vi "Label Example modified3.vi"() -> ()   [LabVIEW 2016]
doc: "This example shows how to label a binary image that contains multiple particles. The labeling process assigns a unique value to all the pixels that belong to a particle. Some processing functions in NI Vision require the input binary image to be labeled."
uses:
  <vilib>/vision/NI_Vision_Development_Module.lvlib
panel:
  out "Labeled":T1(plugin-control)
  out "Region Reports":T2(array[cluster]) {"Mean Value" format="%.2f"; "%" format="%.2f"; "Area (calibrated)" format="%.2f"; "Maximal Value" format="%.2f"; "Minimal Value" format="%.2f"; "Standard Variation" format="%.2f"}
  in  "Stop":bool
  out "Original":T1(plugin-control)
  out "# of Particles found":i32
  in  "Threshold Values":T3(slide)={"Minimum Value"=0.0, "Maximum Value"=65.106384} scale=0.0..255.0
  in  "Connectivity":bool
  # "Tips:\n1) Change the Threshold values to see the Labeled image. \n2) Each distinct particle is labeled with a different pixel value which gives each particle a different color.\n3) Use Binary Palette for Labeled image control"
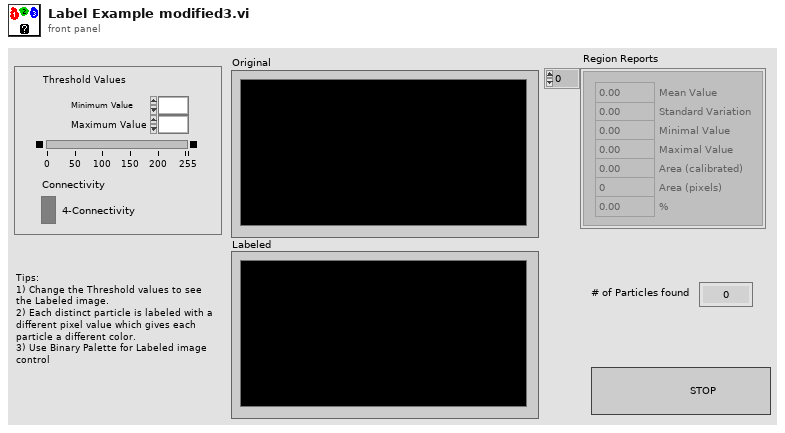
[diagram p1: front panel]
types:
  T1 = typedef "IMAQ Image.ctl" = refnum<image>
  T2 = cluster{"Mean Value":sgl, "Standard Variation":sgl, "Minimal Value":sgl, "Maximal Value":sgl, "Area (calibrated)":sgl, "Area (pixels)":i32, "%":sgl}[]
  T3 = cluster{"Minimum Value":sgl, "Maximum Value":sgl}
  T4 = enum32{"AutoM", "Close", "Dilate", "Erode", "Gradient", "Gradient out", "Gradient in", "Hit miss", "Open", "PClose", "POpen", "Thick", "Thin"}
  T5 = cluster{"Minimum Value":bool, "Maximum Value":bool}
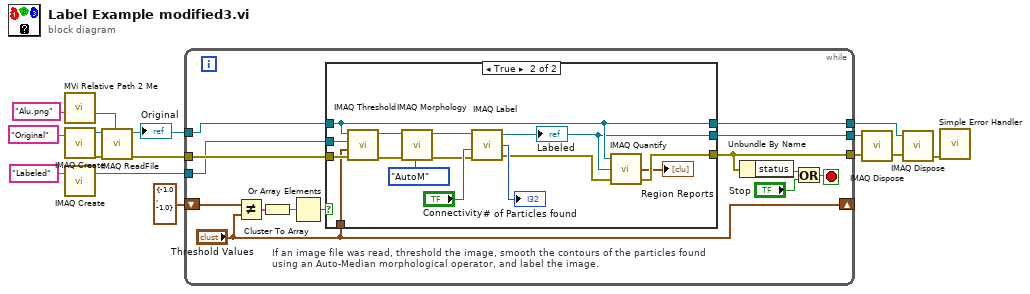
[diagram p0: block diagram]
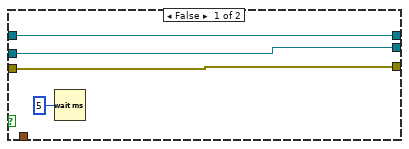
[diagram p2: hidden frame]
diagram:
  n1 = call "MVi Relative Path 2 Me.vi"("Relative Path"="Alu.png" ("name or relative path")) -> ("Appended Dir"=w1:path)  [unwired: 5 in, 1 out]
  n2 = call "IMAQ Create"("Image Name"="Original") -> ("New Image"=w12:T1, "error out"=w13:errorcluster)  [unwired: 4 in]
  n3 = call "IMAQ Create"("Image Name"="Labeled") -> ("New Image"=w9:T1)  [unwired: 4 in, 1 out]
  n4 = call "IMAQ ReadFile"("File Path"=w1, "error in (no error)"=w13, "Image"=w12) -> ("error out"=w10:errorcluster, "Image Out"=w11:T1)  [unwired: 4 in, 3 out]
  "Original" <- w11
  n5 = while {
    tunnel: w11 -> [w29]
    tunnel: w10 -> [w28]
    tunnel: w9 -> [w27]
    shift-right: ["Threshold Values"] -> _
    shift-left: T3 {"Minimum Value"=-1.0, "Maximum Value"=-1.0} ("Threshold Values") -> [w26]
    tunnel: [w16] -> w4
    tunnel: [w17] -> w6
    tunnel: [w18] -> w7
    stop <- w20 stop-if-true
    # "If an image file was read, threshold the image, smooth the contours of the particles found using an Auto-Median morphological operator, and label the image."
    n6 = Not Equal?(x=w26, y="Threshold Values") -> (x != y?=w25:T5)
    n7 = Cluster To Array(cluster=w25) -> (array=w24:bool[])
    n8 = Or Array Elements(Boolean array=w24) -> (logical OR=w23:bool)
    n9 = case shown="True" w23 {
      tunnel: w29 -> [w30 w36]
      tunnel: w28 -> [w32 w43]
      tunnel: w27 -> [w31 w42]
      tunnel: "Threshold Values" -> [_ w39]
      tunnel: [w32 w37] -> w18
      tunnel: [w31 w34] -> w17
      tunnel: [w30 w36] -> w16
      frame False {
        n10 = Wait (ms)(milliseconds to wait=u32 5) -> ()  [unwired: 1 out]
      }
      frame True {
        n11 = call "IMAQ Threshold"("error in (no error)"=w43, "Range"=w39, "Image Dst"=w42, "Image Src"=w36) -> ("error out"=w41:errorcluster, "Image Dst Out"=w47:T1)  [unwired: 6 in]
        n12 = call "IMAQ Morphology"("error in (no error)"=w41, "Operation"=T4."AutoM", "Image Src"=w47) -> ("error out"=w40:errorcluster, "Image Dst Out"=w44:T1)  [unwired: 7 in]
        n13 = call "IMAQ Label"("error in (no error)"=w40, "Connectivity 4/8 (8)"="Connectivity", "Image Src"=w44) -> ("error out"=w38:errorcluster, "Number of Particles"=→"# of Particles found":i32, "Image Dst Out"=w34:T1)  [unwired: 1 in]
        "Labeled" <- w34
        n14 = call "IMAQ Quantify"("error in (no error)"=w38, "Image Mask"=w34, "Image"=w36) -> ("error out"=w37:errorcluster, "Region Reports"=→"Region Reports":T2)  [unwired: 1 out]
      }
    }
    n15 = Unbundle By Name(w18) -> ("status"=w22:bool)
    n16 = Or(x=w22, y="Stop") -> (x .or. y?=w20:bool)
  }
  n17 = call "IMAQ Dispose"("Image"=w6, "error in (no error)"=w7) -> ("error out"=w5:errorcluster)  [unwired: 4 in]
  n18 = call "IMAQ Dispose"("Image"=w4, "error in (no error)"=w5) -> ("error out"=w3:errorcluster)  [unwired: 4 in]
  n19 = call <vilib>:"Simple Error Handler.vi"("error in (no error)"=w3) -> ()  [unwired: 4 in, 5 out]
